vi "Send Launch Views.vi"(8 "error in (no error)":errorcluster, 11 "Message Enqueuer in":refnum<class "Message Enqueuer.lvclass">) -> (0 "error out":errorcluster, 3 "Message Enqueuer out":refnum<class "Message Enqueuer.lvclass">)   [LabVIEW 2015, in "UI Controller.lvlib"]
uses:
  UI Controller.lvlib
  <vilib>/ActorFramework/Message Enqueuer/Message Enqueuer.lvclass
  Views/Side Menu View/Side Menu View/Side Menu.lvclass
  Views/Settings View/Settings View/Settings View.lvclass
  Views/Message Dialog View/Message Dialog View/Message Dialog View.lvclass
  Views/Print View/Print View/Print View.lvclass
  Views/Waiting Dialog View/Waiting Dialog View/Waiting Dialog View.lvclass
  <vilib>/ActorFrameworkMVC/Abstract Controller/Abstract Controller Messages/Launch View Msg/Launch View Msg.lvclass/Launch View Msg.ctl
  <vilib>/ActorFramework/Message Enqueuer/Message Enqueuer.lvclass/Message Enqueuer.ctl
  <vilib>/ActorFramework/Message Enqueuer/Enqueue.vi
  <vilib>/ActorFramework/Message Priority Queue/Priority Enqueue.vi
  <vilib>/ActorFrameworkMVC/Abstract Controller/Abstract Controller Messages/Launch View Msg/Launch View Msg.lvclass
panel:
  # "NOTICE -- YOU MUST LEAVE THIS NOTICE IN PLACE.\n\nCopyright (c) 2015, LIANG LIU Shawn.Liu.cn@gmail.com\nAll rights reserved.\n\nRedistribution and use in source and binary forms, with or without modification, are permitted provided that the following conditions are met:\n-Redistributions of source code must retain the above copyright notice, this list of conditions and the following disclaimer.\n-Redistributions in binary form must reproduce the above copyright notice, this list of conditions and the following disclaimer in the documentation and/or other materials provided with the distribution.\n-Neither the name of the eLp nor the names of its contributors may be used to endorse or promote products derived from this software without specific prior written permission.\n\nTHIS SOFTWARE IS PROVIDED BY THE COPYRIGHT HOLDERS AND CONTRIBUTORS \"AS IS\" AND ANY EXPRESS OR IMPLIED WARRANTIES, INCLUDING, BUT NOT LIMITED TO, THE IMPLIED WARRANTIES OF MERCHANTABILITY AND FITNESS FOR A PARTICULAR PURPOSE ARE DISCLAIMED. IN NO EVENT SHALL THE COPYRIGHT HOLDER OR CONTRIBUTORS BE LIABLE FOR ANY DIRECT, INDIRECT, INCIDENTAL, SPECIAL, EXEMPLARY, OR CONSEQUENTIAL DAMAGES (INCLUDING, BUT NOT LIMITED TO, PROCUREMENT OF SUBSTITUTE GOODS OR SERVICES; LOSS OF USE, DATA, OR PROFITS; OR BUSINESS INTERRUPTION) HOWEVER CAUSED AND ON ANY THEORY OF LIABILITY, WHETHER IN CONTRACT, STRICT LIABILITY, OR TORT (INCLUDING NEGLIGENCE OR OTHERWISE) ARISING IN ANY WAY OUT OF THE USE OF THIS SOFTWARE, EVEN IF ADVISED OF THE POSSIBILITY OF SUCH DAMAGE."
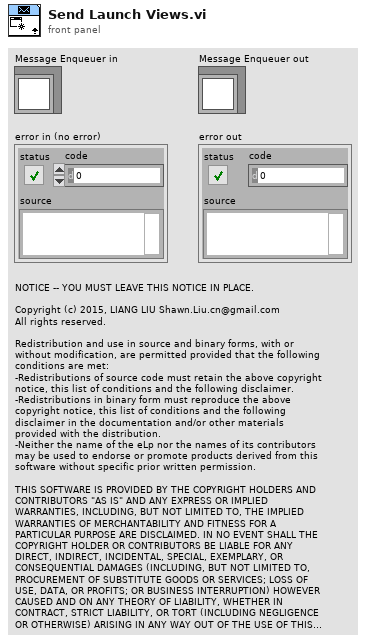
[diagram p1: front panel]
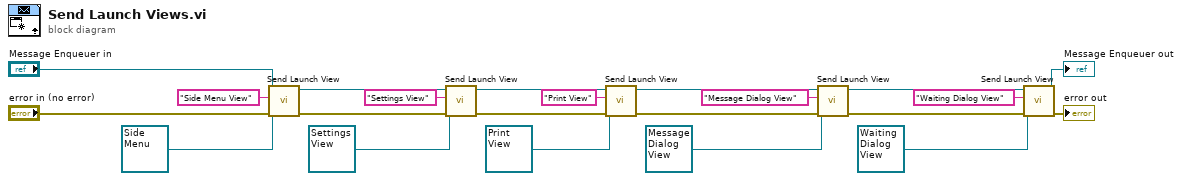
[diagram p0: block diagram]
diagram:
  n1 = call <vilib>:"Send Launch View.vi"("error in (no error)"="error in (no error)", "View"=refnum<class "Side Menu.lvclass"> refnum ("Side Menu.lvlib:Side Menu.lvclass"), "View Name"="Side Menu View", "Message Enqueuer"="Message Enqueuer in") -> ("error out"=w17:errorcluster, "Message Enqueuer out"=w10:refnum<class "Message Enqueuer.lvclass">)  [unwired: 6 in]
  n2 = call <vilib>:"Send Launch View.vi"("error in (no error)"=w17, "View"=refnum<class "Settings View.lvclass"> refnum ("Settings Flyout.lvlib:Settings Flyout.lvclass"), "View Name"="Settings View", "Message Enqueuer"=w10) -> ("error out"=w18:errorcluster, "Message Enqueuer out"=w11:refnum<class "Message Enqueuer.lvclass">)  [unwired: 6 in]
  n3 = call <vilib>:"Send Launch View.vi"("error in (no error)"=w18, "View"=refnum<class "Print View.lvclass"> refnum ("Print Flyout.lvlib:Print Flyout.lvclass"), "View Name"="Print View", "Message Enqueuer"=w11) -> ("error out"=w19:errorcluster, "Message Enqueuer out"=w16:refnum<class "Message Enqueuer.lvclass">)  [unwired: 6 in]
  n4 = call <vilib>:"Send Launch View.vi"("error in (no error)"=w19, "View"=refnum<class "Message Dialog View.lvclass"> refnum ("Message Dialog.lvlib:Message Dialog.lvclass"), "View Name"="Message Dialog View", "Message Enqueuer"=w16) -> ("error out"=w22:errorcluster, "Message Enqueuer out"=w5:refnum<class "Message Enqueuer.lvclass">)  [unwired: 6 in]
  n5 = call <vilib>:"Send Launch View.vi"("error in (no error)"=w22, "View"=refnum<class "Waiting Dialog View.lvclass"> refnum ("Waiting Dialog View.lvlib:Waiting Dialog.lvclass"), "View Name"="Waiting Dialog View", "Message Enqueuer"=w5) -> ("error out"=→"error out":errorcluster, "Message Enqueuer out"=→"Message Enqueuer out":refnum<class "Message Enqueuer.lvclass">)  [unwired: 6 in]
